vi "LEP_RV_CompoundXMLFileName.vi"(11 "Project file path":path) -> (3 "Path for XML generated file":path)   [LabVIEW 2011]
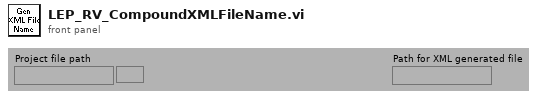
[diagram p1: front panel]
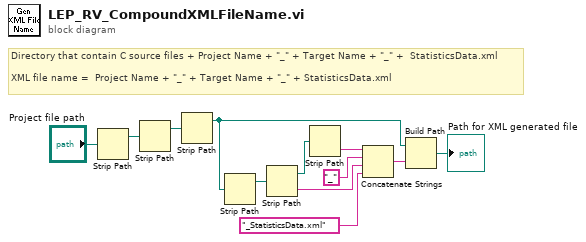
[diagram p0: block diagram]
diagram:
  # "Directory that contain C source files + Project Name + \"_\" + Target Name + \"_\" +  StatisticsData.xml\n\nXML file name =  Project Name + \"_\" + Target Name + \"_\" + StatisticsData.xml"
  n1 = Strip Path(path="Project file path") -> (stripped path=w10:path)  [unwired: 1 out]
  n2 = Strip Path(path=w10) -> (stripped path=w9:path)  [unwired: 1 out]
  n3 = Strip Path(path=w9) -> (stripped path=w3:path)  [unwired: 1 out]
  n4 = Strip Path(path=w3) -> (stripped path=w8:path)  [unwired: 1 out]
  n5 = Strip Path(path=w8) -> (stripped path=w7:path, name=w6:string)
  n6 = Strip Path(path=w7) -> (name=w4:string)  [unwired: 1 out]
  n7 = Concatenate Strings(w4, "_" ("string"), w6, "_StatisticsData.xml") -> (w2:string)
  n8 = Build Path(base path=w3, name or relative path=w2) -> (appended path=→"Path for XML generated file":path)
